vi "XIPIN_Image_Edge_Enhancement_2_0.vi"   [LabVIEW 2017]
doc: "The Xilinx Edge Enhancement LogiCORE provides edge enhancement of each frame of video data being processed. The core provides a set of standard Sobel and Laplacian filters with programmable, edge adaptive gain settings to adjust the strength of the edge enhancement effect.\n------------------------------------\n<b>Need License</b> : Yes"
uses:
  <vilib>/rvi/XilinxIP/XIPIN_XNode/niFpgaXIPIN.xnode
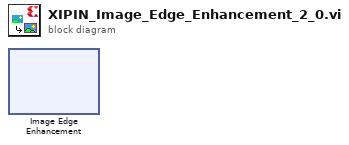
[diagram p0: block diagram]
diagram:
  n1 = xnode ("Image Edge Enhancement")() -> ()
